vi "scan2d_plot_data.vi"(8 "error in (no error)":errorcluster, 11 "scan_panel in":refnum<class "scan_2d.lvclass">) -> (0 "error out":errorcluster, 3 "scan_panel out":refnum<class "scan_2d.lvclass">)   [LabVIEW 2015, in "scan_2d.lvclass"]
uses:
  scan_2d.lvclass
  UI/panel_class/panel.lvclass/panel.ctl
  scan_2d.lvclass/scan_2d.ctl
  scan_2d_hdf5_log/scan_2d_hdf5_log.lvclass
  UI/panel_class/panel.lvclass
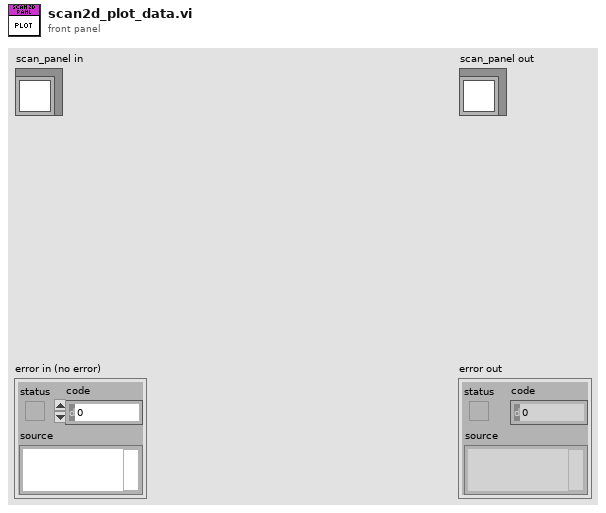
[diagram p1: front panel]
types:
  T1 = typedef "ui_user_events.ctl" = cluster{"update_xy_graph":refnum<user-event>, "update_graph":refnum<user-event>, "update_chart":refnum<user-event>, "update_map":refnum<user-event>, "event_loop_stop":refnum<user-event>, "keep_map":refnum<user-event>}
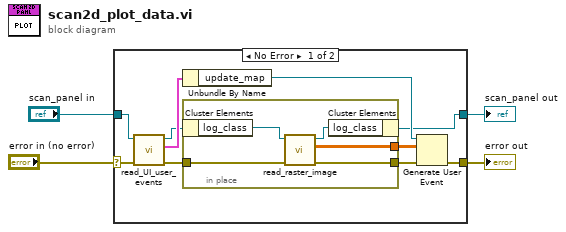
[diagram p0: block diagram]
diagram:
  n1 = case shown="No Error" "error in (no error)" {
    selector: "error in (no error)" -> [w11 w21]
    tunnel: [w6 w21] -> w3
    tunnel: [w8 w20] -> w1
    tunnel: "scan_panel in" -> [w12 w20]
    frame No Error {
      n2 = call "read_UI_user_events.vi"("error in (no error)"=w11, "panel in"=w12) -> ("error out"=w10:errorcluster, "ui_user_events"=w14:T1, "panel out"=w5:refnum<class "scan_2d.lvclass">)  [unwired: 7 in]
      n3 = Unbundle By Name(w14) -> ("update_map"=w13:refnum<user-event>)
      n4 = in-place {
        in-place-border: w10 -> [w16]
        in-place-border: [w17] -> w9
        in-place-border: [w15] -> w7
        n5 = in-place-cluster #1(w5) -> ("log_class"=w19:refnum<class "scan_2d_hdf5_log.lvclass">)
        n6 = call-dynamic "read_raster_image.vi"("error in (no error)"=w16, "scan_2d_hdf5_log in"=w19) -> ("error out"=w15:errorcluster, "raster_image"=w17:dbl[][], "scan_2d_hdf5_log out"=w18:refnum<class "scan_2d_hdf5_log.lvclass">)  [unwired: 7 in]
        n7 = in-place-cluster #1("log_class"=w18) -> (w8:refnum<class "scan_2d.lvclass">)
      }
      n8 = Generate User Event(user event=w13, event data cluster=w9, error in=w7) -> (error out=w6:errorcluster)  [unwired: 1 in, 1 out]
    }
    frame Error {
    }
  }
  "error out" <- w3
  "scan_panel out" <- w1
